vi "Initialize Icon Decorator.vi"(8 "error in (no error)":errorcluster, 11 "Execution UI in":refnum<class "Execution UI.lvclass">) -> (0 "error out":errorcluster, 3 "Execution UI Out":refnum<class "Execution UI.lvclass">)   [LabVIEW 2020, in "Execution UI.lvclass"]
uses:
  Execution UI.lvclass
  Execution UI.lvclass/Execution UI.ctl
  Icon Decorator/Icon Decorator.lvclass
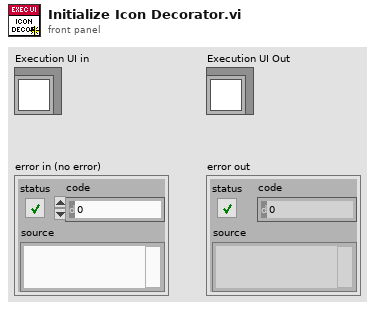
[diagram p1: front panel]
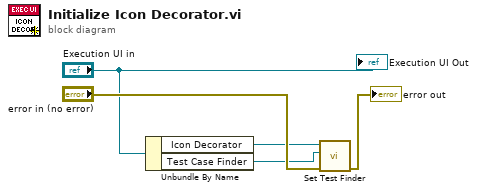
[diagram p0: block diagram]
diagram:
  n1 = Unbundle By Name("Execution UI in") -> ("Icon Decorator"=w2:refnum<class "Icon Decorator.lvclass">, "Test Case Finder"=w3:refnum<class "Test Finder.lvclass">)
  n2 = call "Set Test Finder.vi"("error in (no error)"="error in (no error)", "Report Generator"=w3, "Icon Decorator In"=w2) -> ("error out"=→"error out":errorcluster)  [unwired: 7 in, 1 out]
  "Execution UI Out" <- "Execution UI in"
